vi "POST.vi"(7 "LabVIEW Web Service Request":refnum<class "Web Request.lvclass">) -> ()   [LabVIEW 2015]
uses:
  <vilib>/wsapi/Web Request.lvclass
panel:
  out "session ID cookie":string
  # "Use the Web Service Request input terminal to call the VIs on the Web Services palette. Do not remove it from the connector pane unless you don't need access to the palette."
  # "Each additional control wired to the connector pane will be available as an input in the URL. To include an indicator in terminal-mode output (the default setting), it must also be wired to the connector pane."
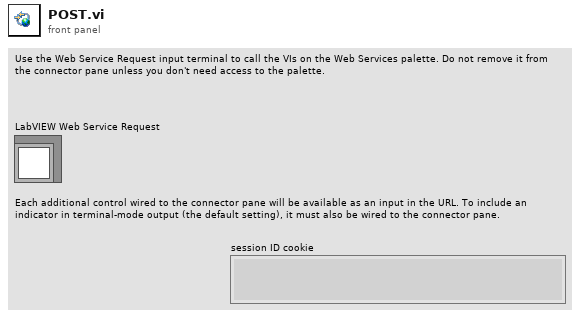
[diagram p1: front panel]
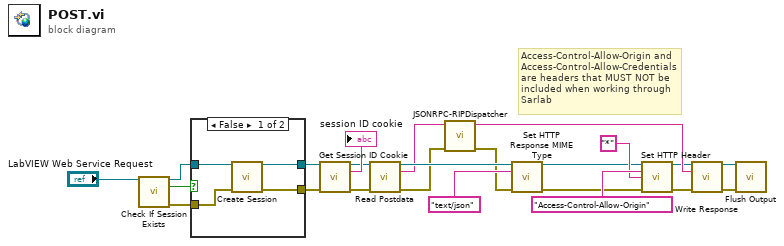
[diagram p0: block diagram]
diagram:
  # "Access-Control-Allow-Origin and\nAccess-Control-Allow-Credentials\nare headers that MUST NOT be\nincluded when working through\nSarlab"
  n1 = call <vilib>:"Check If Session Exists.vi"("LabVIEW Web Service Request"="LabVIEW Web Service Request") -> ("LabVIEW Web Service Request out"=w23:refnum<class "Web Request.lvclass">, "session exists?"=w22:bool, "error out"=w20:errorcluster)  [unwired: 12 in]
  n2 = case shown="False" w22 {
    tunnel: w23 -> [w27 w29]
    tunnel: [w26 w29] -> w21
    tunnel: w20 -> [w25 w28]
    tunnel: [w24 w28] -> w19
    frame False {
      n3 = call <vilib>:"Create Session.vi"("LabVIEW Web Service Request"=w27, "error in (no error)"=w25) -> ("LabVIEW Web Service Request out"=w26:refnum<class "Web Request.lvclass">, "error out"=w24:errorcluster)  [unwired: 11 in, 1 out]
    }
    frame True {
    }
  }
  n4 = call <vilib>:"Get Session ID Cookie.vi"("LabVIEW Web Service Request"=w21, "error in (no error)"=w19) -> ("LabVIEW Web Service Request out"=w17:refnum<class "Web Request.lvclass">, "session ID cookie"=→"session ID cookie":string, "error out"=w16:errorcluster)  [unwired: 11 in]
  n5 = call <vilib>:"Read Postdata.vi"("LabVIEW Web Service Request"=w17, "error in (no error)"=w16) -> ("LabVIEW Web Service Request out"=w11:refnum<class "Web Request.lvclass">, "postdata"=w10:string, "error out"=w9:errorcluster)  [unwired: 11 in]
  n6 = call "JSONRPC-RIPDispatcher.vi"("error in"=w9, "input string"=w10) -> ("error out"=w7:errorcluster, "response"=w8:string)  [unwired: 8 in]
  n7 = call <vilib>:"Set HTTP Response MIME Type.vi"("LabVIEW Web Service Request"=w11, "MIME type (text/html)"="text/json" ("header"), "error in (no error)"=w7) -> ("LabVIEW Web Service Request out"=w3:refnum<class "Web Request.lvclass">, "error out"=w4:errorcluster)  [unwired: 11 in]
  n8 = call <vilib>:"Set HTTP Header.vi"("LabVIEW Web Service Request"=w3, "header"="Access-Control-Allow-Origin", "header value"="*", "error in (no error)"=w4) -> ("LabVIEW Web Service Request out"=w2:refnum<class "Web Request.lvclass">, "error out"=w1:errorcluster)  [unwired: 10 in]
  n9 = call <vilib>:"Write Response.vi"("LabVIEW Web Service Request"=w2, "response string"=w8, "error in (no error)"=w1) -> ("LabVIEW Web Service Request out"=w14:refnum<class "Web Request.lvclass">, "error out"=w13:errorcluster)  [unwired: 11 in]
  n10 = call <vilib>:"Flush Output.vi"("LabVIEW Web Service Request"=w14, "error in (no error)"=w13) -> ()  [unwired: 12 in, 2 out]
